vi "Main Scan Processor Status.vi"() -> ()   [LabVIEW 2017]
panel:
  out "Table Stage Processor":bool
  out "Busy":bool
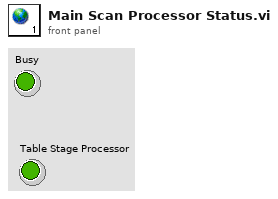
[diagram p1: front panel]
diagram:
